vi "subvi in roop.vi"(8 "error in":errorcluster, 9 "Option":T1, 10 "Encoding?":T2=enum."UTF-16 LE", 11 "Path in":path) -> (0 "error out":errorcluster, 2 "UTF-8 String":string, 3 "Path out":path)   [LabVIEW 2011]
uses:
  Text Encoding Format.ctl
  Read Write AU Text File option.ctl
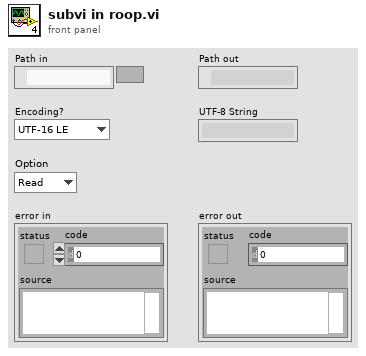
[diagram p1: front panel]
types:
  T1 = typedef "Read Write AU Text File option.ctl" = enum16{"Read", "Write"}
  T2 = typedef "Text Encoding Format.ctl" = enum8{"ASCII", "UTF-8", "UTF-16 LE", "UTF-16 BE"}
  T3 = enum16{"open", "replace", "create", "open or create", "replace or create", "replace or create with confirmation"}
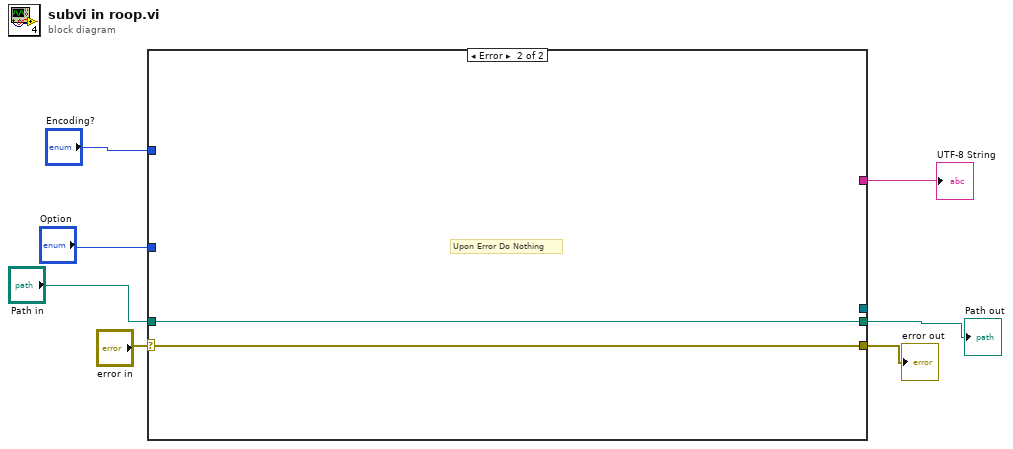
[diagram p0: block diagram]
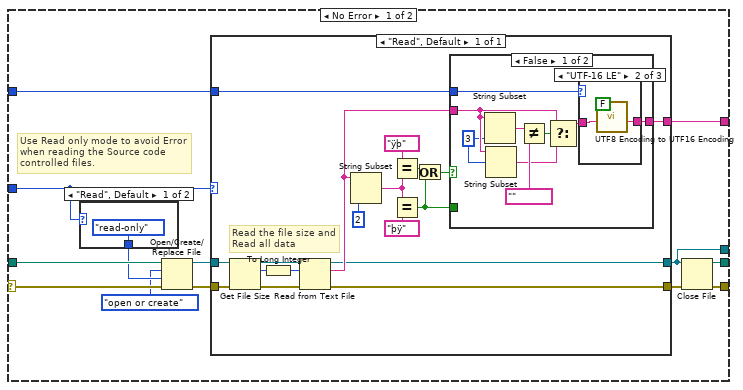
[diagram p2: hidden frame]
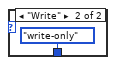
[diagram p3: hidden frame]
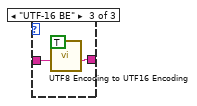
[diagram p5: hidden frame]
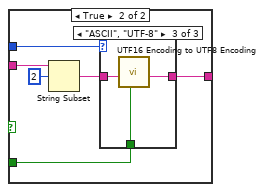
[diagram p6: hidden frame]
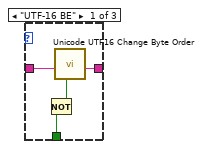
[diagram p7: hidden frame]
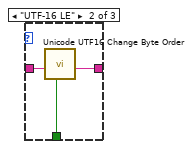
[diagram p8: hidden frame]
diagram:
  n1 = case shown="Error" "error in" {
    selector: "error in" -> [w18 w74]
    tunnel: [w10 w74] -> w5
    tunnel: "Path in" -> [w19 w73]
    tunnel: [w20 _] -> w6
    tunnel: [w12 w73] -> w4
    tunnel: "Option" -> [w8 _]
    tunnel: "Encoding?" -> [w13 _]
    tunnel: [w9 _] -> _
    frame No Error {
      # "Use Read only mode to avoid Error \nwhen reading the Source code \ncontrolled files."
      n2 = case shown="\"Read\", Default" w8 {
        tunnel: [enum16{"read/write", "read-only", "write-only"}."read-only" ("access (0:read/write)") enum16{"read/write", "read-only", "write-only"}."write-only" ("access (0:read/write)")] -> w17
        frame "Read", Default {
        }
        frame "Write" {
        }
      }
      n3 = Open/Create/Replace File(file path (use dialog)=w19, error in=w18, operation (0:open)=T3."open or create", access (0:read/write)=w17) -> (refnum out=w16:refnum<file>, error out=w15:errorcluster)  [unwired: 2 in, 1 out]
      n4 = case shown="\"Read\", Default" w8 {
        tunnel: [w33] -> w20
        tunnel: [w31] -> w9
        tunnel: [w30] -> w11
        tunnel: w16 -> [w28]
        tunnel: w15 -> [w26]
        tunnel: w13 -> [w29]
        frame "Read", Default {
          # "Read the file size and \nRead all data"
          n5 = Get File Size(file=w28, error in=w26) -> (refnum out=w27:refnum<file>, size (in bytes)=w24:i64, 0:w25:errorcluster)
          n6 = To Long Integer(number=w24) -> (32bit integer=w23:i32)
          n7 = Read from Text File(file (use dialog)=w27, count=w23, error in=w25) -> (refnum out=w31:refnum<file>, text=w32:string, error out=w30:errorcluster)  [unwired: 1 in, 1 out]
          n8 = String Subset(string=w32, length (rest)=2 ("length (rest)")) -> (substring=w38:string)  [unwired: 1 in]
          n9 = Equal?(x="ÿþ" ("text 2"), y=w38) -> (x = y?=w35:bool)
          n10 = Equal?(x=w38, y="þÿ" ("text 2")) -> (x = y?=w36:bool)
          n11 = Or(x=w35, y=w36) -> (x .or. y?=w34:bool)
          n12 = case shown="False" w34 {
            tunnel: w32 -> [w45 w61]
            tunnel: [w42 w60] -> w33
            tunnel: w36 -> [_ w58]
            tunnel: w29 -> [w43 w57]
            frame False {
              w44 = 3 ("offset (0)")
              n13 = String Subset(string=w45, length (rest)=w44) -> (substring=w48:string)  [unwired: 1 in]
              n14 = String Subset(string=w45, offset (0)=w44) -> (substring=w46:string)  [unwired: 1 out]
              n15 = Not Equal?(x=w48, y="﻿" ("text 2")) -> (x != y?=w47:bool)
              n16 = Select(t=w45, s=w47, f=w46) -> (s? t:f=w41:string)
              n17 = case shown="\"UTF-16 LE\"" w43 {
                tunnel: [w50 w52 w55] -> w42
                tunnel: w41 -> [w50 w53 w56]
                frame "ASCII", "UTF-8" {
                }
                frame "UTF-16 LE" {
                  n18 = call "UTF8 Encoding to UTF16 Encoding.vi"("Big Endian?"=FALSE, "UTF-8 String"=w53) -> ("UTF-16 String"=w52:string)  [unwired: 8 in, 1 out]
                }
                frame "UTF-16 BE" {
                  n19 = call "UTF8 Encoding to UTF16 Encoding.vi"("Big Endian?"=TRUE, "UTF-8 String"=w56) -> ("UTF-16 String"=w55:string)  [unwired: 8 in, 1 out]
                }
              }
            }
            frame True {
              n20 = String Subset(string=w61, offset (0)=2) -> (substring=w59:string)  [unwired: 1 out]
              n21 = case shown="\"ASCII\", \"UTF-8\"" w57 {
                tunnel: [w64 w68 w71] -> w60
                tunnel: w59 -> [w65 w69 w72]
                tunnel: w58 -> [w66 w67 w70]
                frame "UTF-16 BE" {
                  n22 = Not(x=w66) -> (.not. x?=w63:bool)
                  n23 = call "Unicode UTF16 Change Byte Order.vi"("Change BO?"=w63, "UTF-16 String In"=w65) -> ("UTF-16 String Out"=w64:string)  [unwired: 8 in, 1 out]
                }
                frame "UTF-16 LE" {
                  n24 = call "Unicode UTF16 Change Byte Order.vi"("Change BO?"=w67, "UTF-16 String In"=w69) -> ("UTF-16 String Out"=w68:string)  [unwired: 8 in, 1 out]
                }
                frame "ASCII", "UTF-8" {
                  n25 = call "UTF16 Encoding to UTF8 Encoding.vi"("Big Endian?"=w70, "UTF-16 String"=w72) -> ("UTF-8 String"=w71:string)  [unwired: 8 in, 1 out]
                }
              }
            }
          }
        }
      }
      n26 = Close File(refnum=w9, error in=w11) -> (path=w12:path, error out=w10:errorcluster)
    }
    frame Error {
      # "Upon Error Do Nothing"
    }
  }
  "UTF-8 String" <- w6
  "error out" <- w5
  "Path out" <- w4
